vi "例8.3 利用DAQ助手连续模入.vi"() -> ()   [LabVIEW 2017]
panel:
  out "波形图":dynamicdata(graph)
  out "波形图表":dynamicdata(graph)
  in  "stop (F)":bool caption="停止(F)"
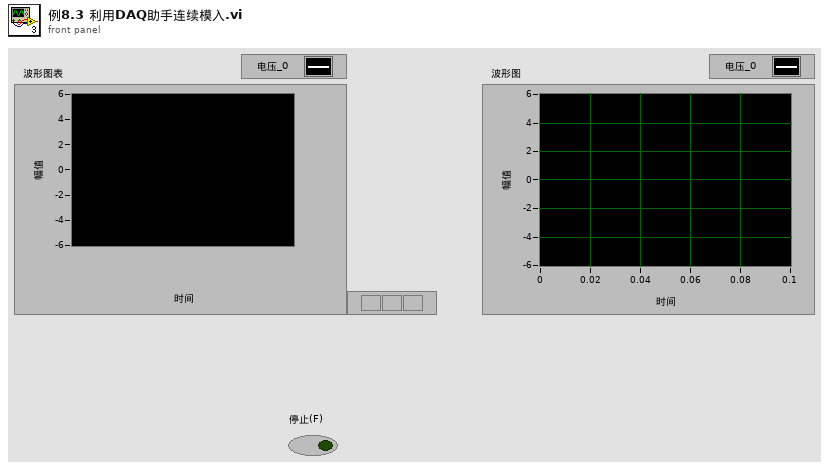
[diagram p1: front panel]
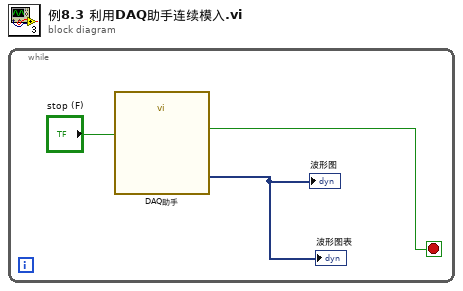
[diagram p0: block diagram]
diagram:
  n1 = while {
    stop <- w2 stop-if-true
    n2 = call "DAQ助手"("stop (F)"="stop (F)") -> ("data"=→"波形图" →"波形图表":dynamicdata, "stopped"=w2:bool)  [unwired: 15 in, 2 out]
  }
